vi "LookAhead.vi"(7 "error in (no error)":errorcluster, 9 "Index":i32, 10 "JSON String":string) -> (0 "error out":errorcluster, 1 "TOKEN":T1, 2 "Index Passthrough":i32, 3 "JSON String Passthrough":string)   [LabVIEW 2010, in "i3-json.lvlib"]
doc: "Use this template to build a VI to use as a subVI."
uses:
  i3-json.lvlib
  Token.ctl
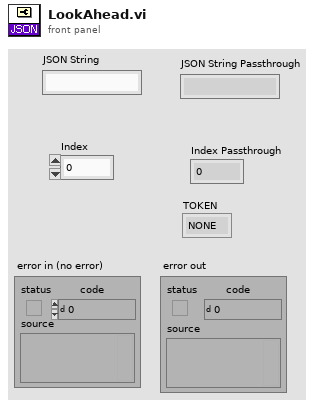
[diagram p1: front panel]
types:
  T1 = typedef "i3-json.lvlib/Token.ctl" = enum16{"NONE", "CURLY_OPEN", "CURLY_CLOSE", "SQUARED_OPEN", "SQUARED_CLOSE", "COLON", "COMMA", "STRING", "NUMBER", "TRUE", "FALSE", "NULL"}
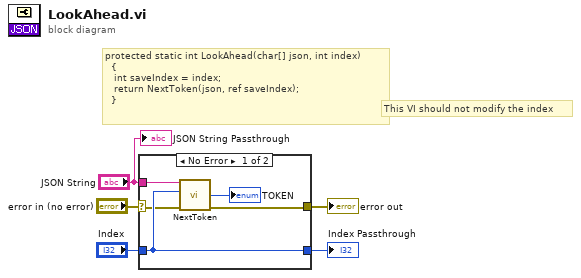
[diagram p0: block diagram]
diagram:
  # "This VI should not modify the index"
  # "protected static int LookAhead(char[] json, int index)\n\t\t{\n\t\t\tint saveIndex = index;\n\t\t\treturn NextToken(json, ref saveIndex);\n\t\t}"
  n1 = case shown="No Error" "error in (no error)" {
    selector: "error in (no error)" -> [w8 w12]
    tunnel: [w7 w12] -> w4
    tunnel: "JSON String" -> [w10 _]
    tunnel: [w9 w11] -> w2
    tunnel: "Index" -> [w9 w11]
    frame No Error {
      n2 = call "NextToken.vi"("error in (no error)"=w8, "Index In"=w9, "JSON String"=w10) -> ("error out"=w7:errorcluster, "TOKEN"=→"TOKEN":T1)  [unwired: 4 in, 2 out]
    }
    frame Error {
    }
  }
  "error out" <- w4
  "Index Passthrough" <- w2
  "JSON String Passthrough" <- "JSON String"
